vi "test buzy Q.vi"() -> ()   [LabVIEW 2014]
panel:
  in  "Boolean":bool
  out "# elements in queue":i32
  in  "stop":bool
  out "Buzy10":i32
  out "Buzy500":i32
  out "Buzy1000":i32
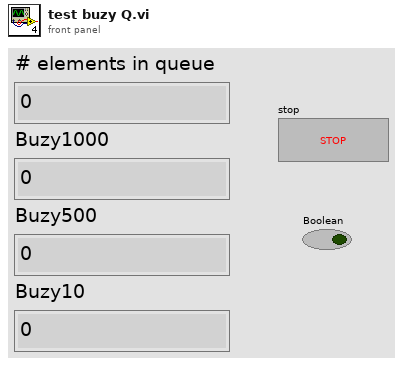
[diagram p1: front panel]
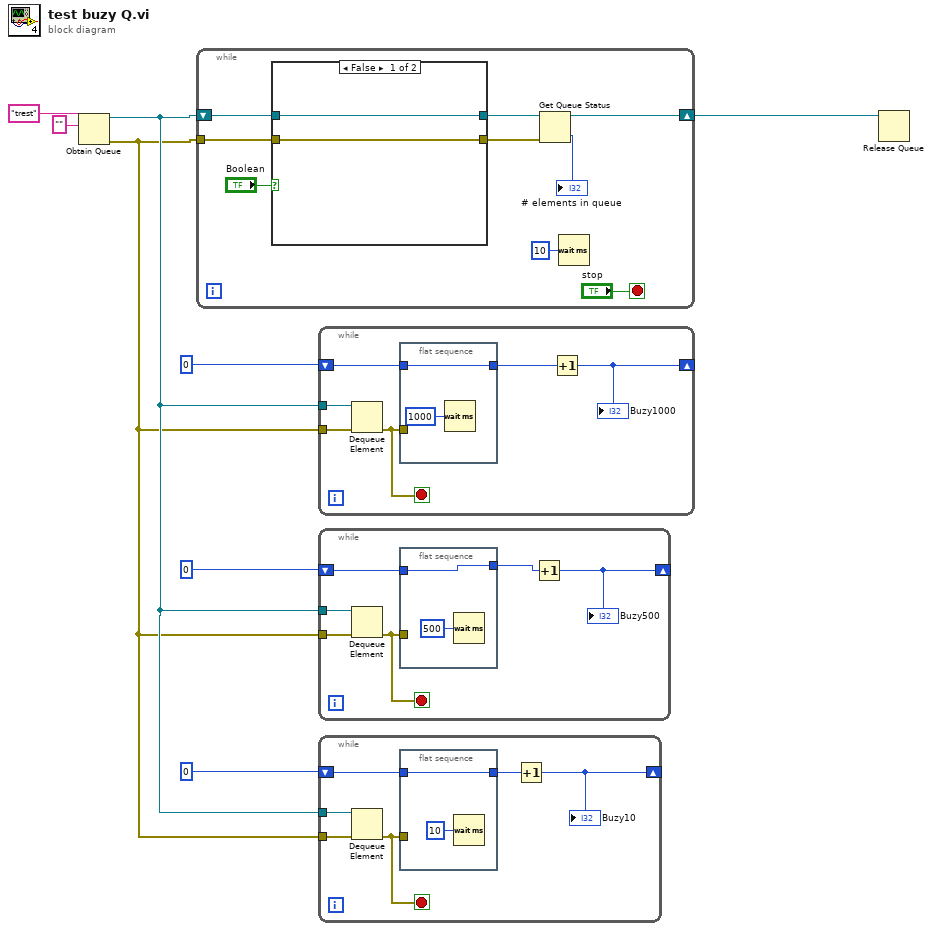
[diagram p0: block diagram]
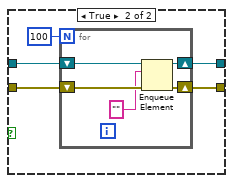
[diagram p2: hidden frame]
diagram:
  n1 = Obtain Queue(name (unnamed)="trest", element data type="") -> (queue out=w3:refnum<queue>, error out=w2:errorcluster)  [unwired: 3 in, 1 out]
  n2 = while {
    tunnel: w2 -> [w14]
    shift-right: [w12] -> w1
    shift-left: w3 -> [w15]
    stop <- "stop" stop-if-true
    n3 = case shown="False" "Boolean" {
      tunnel: w15 -> [w18 w24]
      tunnel: w14 -> [w19 w23]
      tunnel: [w18 w22] -> w13
      tunnel: [w19 w21] -> w11
      frame False {
      }
      frame True {
        n4 = for {
          N: 100 -> [_]
          shift-right: [w27] -> w22
          shift-left: w24 -> [w29]
          shift-right: [w26] -> w21
          shift-left: w23 -> [w28]
          n5 = Enqueue Element(queue=w29, element="", error in (no error)=w28) -> (queue out=w27:refnum<queue>, error out=w26:errorcluster)  [unwired: 1 in, 1 out]
        }
      }
    }
    n6 = Get Queue Status(queue=w13, error in (no error)=w11) -> (queue out=w12:refnum<queue>, # elements in queue=→"# elements in queue":i32)  [unwired: 1 in, 6 out]
    n7 = Wait (ms)(milliseconds to wait=u32 10) -> ()  [unwired: 1 out]
  }
  n8 = while {
    tunnel: w3 -> [w35]
    tunnel: w2 -> [w34]
    shift-right: [w33] -> _
    shift-left: 0 -> [w30]
    stop <- w32 stop-if-true
    n9 = Dequeue Element(queue=w35, error in (no error)=w34) -> (error out=w32:errorcluster)  [unwired: 1 in, 3 out]
    n10 = flat-sequence {
      tunnel: w32 -> [_]
      tunnel: [w36] -> w31
      tunnel: w30 -> [w36]
      frame #0 {
        n11 = Wait (ms)(milliseconds to wait=u32 1000) -> ()  [unwired: 1 out]
      }
    }
    n12 = Increment(x=w31) -> (x+1=w33:i32)
    "Buzy1000" <- w33
  }
  n13 = while {
    tunnel: w3 -> [w43]
    tunnel: w2 -> [w42]
    shift-right: [w41] -> _
    shift-left: 0 -> [w38]
    stop <- w40 stop-if-true
    n14 = Dequeue Element(queue=w43, error in (no error)=w42) -> (error out=w40:errorcluster)  [unwired: 1 in, 3 out]
    n15 = flat-sequence {
      tunnel: w40 -> [_]
      tunnel: [w44] -> w39
      tunnel: w38 -> [w44]
      frame #0 {
        n16 = Wait (ms)(milliseconds to wait=u32 500) -> ()  [unwired: 1 out]
      }
    }
    n17 = Increment(x=w39) -> (x+1=w41:i32)
    "Buzy500" <- w41
  }
  n18 = while {
    tunnel: w3 -> [w51]
    tunnel: w2 -> [w50]
    shift-right: [w49] -> _
    shift-left: 0 -> [w46]
    stop <- w48 stop-if-true
    n19 = Dequeue Element(queue=w51, error in (no error)=w50) -> (error out=w48:errorcluster)  [unwired: 1 in, 3 out]
    n20 = flat-sequence {
      tunnel: w48 -> [_]
      tunnel: [w52] -> w47
      tunnel: w46 -> [w52]
      frame #0 {
        n21 = Wait (ms)(milliseconds to wait=u32 10) -> ()  [unwired: 1 out]
      }
    }
    n22 = Increment(x=w47) -> (x+1=w49:i32)
    "Buzy10" <- w49
  }
  n23 = Release Queue(queue=w1) -> ()  [unwired: 2 in, 3 out]
